vi "Write U64.vi"(8 "error in (no error)":errorcluster, 9 "Timeout (ms)":i32, 10 "Data":u64, 11 "CIFTag in":refnum<class "CIF_NIChn_U64.lvclass">) -> (0 "error out":errorcluster, 1 "timed out?":bool, 3 "CIFTag out":refnum<class "CIF_NIChn_U64.lvclass">)   [LabVIEW 2021, in "CIF_NIChn_U64.lvclass"]
uses:
  CIF_NIChn_U64.lvclass
  D:/dev/Packages/Channel_Manager/src/CIF_NIChn/NIChn/CIF_NIChn.lvclass
  NIChn/CIF_NIChn.lvclass/CIF_NIChn.ctl
  CIF_NIChn_U64.lvclass/CIF_NIChn_U64.ctl
  e6e5dc56-0fe0-434b-816e-55c2e61471c2.vi
  e6e5dc56-0fe0-434b-816e-55c2e61471c2.vi/4bc1c15b-36ab-481f-b8dd-c64075ce723a.vi
  e6e5dc56-0fe0-434b-816e-55c2e61471c2.vi/d83cb72b-7713-41fc-a3d1-682de79cf574.vi
  <vilib>/CIF Foundation/CIF Channels/CIFChannels/SubVIs/Get dll Path.vi
  NIChn/CIF_NIChn.lvclass
  D:/dev/Packages/Channel_Manager/src/CIFChannels/CIFChannels.lvclass
  D:/dev/Packages/Channel_Manager/src/CIF_NIChn/U64/CIF_NIChn_U64.lvclass
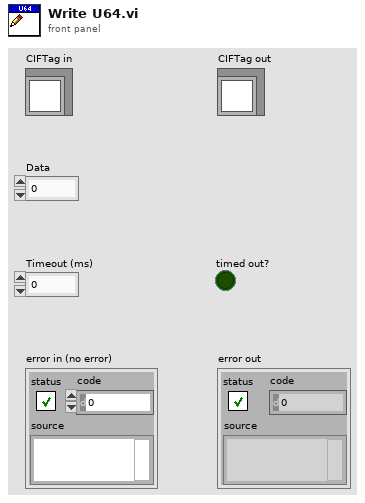
[diagram p1: front panel]
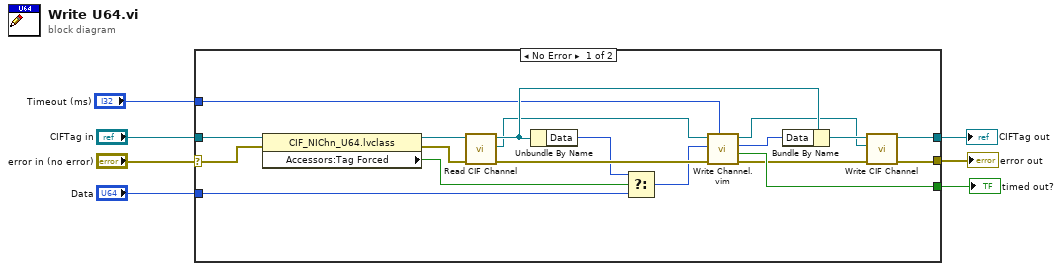
[diagram p0: block diagram]
diagram:
  n1 = case shown="No Error" "error in (no error)" {
    selector: "error in (no error)" -> [w14 w28]
    tunnel: [w20 w28] -> w6
    tunnel: [w22 w27] -> w4
    tunnel: "CIFTag in" -> [w15 w27]
    tunnel: "Data" -> [w11 _]
    tunnel: [w26 _] -> w2
    tunnel: "Timeout (ms)" -> [w17 _]
    frame No Error {
      n2 = property class="CIF_NIChn_U64.lvclass"(reference=w15, error in=w14) -> (reference out=w13:refnum<class "CIF_NIChn_U64.lvclass">, error out=w8:errorcluster, "Accessors:Tag Forced"=w12:bool)
      n3 = call "Read CIF Channel.vi"("error in (no error)"=w8, "CIFTag in"=w13) -> ("error out"=w24:errorcluster, "CIF Channel"=w19:refnum<k21>, "CIFTag out"=w25:refnum<class "CIF_NIChn_U64.lvclass">)  [unwired: 7 in]
      n4 = Unbundle By Name(w25) -> ("Data"=w10:u64)
      n5 = Select(t=w10, s=w12, f=w11) -> (s? t:f=w9:u64)
      n6 = call "Write Channel.vim"("Timeout (ms)"=w17, "error in"=w24, "Data in"=w9, "CIF Channel in"=w19) -> ("error out"=w21:errorcluster, "Timed out?"=w26:bool, "Data out"=w16:u64, "CIF Channel out"=w18:refnum<k21>)  [unwired: 4 in]
      n7 = Bundle By Name(cluster=w25, "Data"=w16) -> (w23:refnum<class "CIF_NIChn_U64.lvclass">)
      n8 = call "Write CIF Channel.vi"("error in (no error)"=w21, "CIF Channel"=w18, "CIFTag in"=w23) -> ("error out"=w20:errorcluster, "CIFTag out"=w22:refnum<class "CIF_NIChn_U64.lvclass">)  [unwired: 7 in]
    }
    frame Error {
    }
  }
  "error out" <- w6
  "CIFTag out" <- w4
  "timed out?" <- w2
